vi "UpdateCfgIni.vi"(8 "error in":errorcluster, 10 "contentArray":string[](array[string]), 11 "iniCfgRefnumIn":refnum<file>) -> (0 "error out":errorcluster, 3 "iniCfgRefnumOut":refnum<file>)   [LabVIEW 2010]
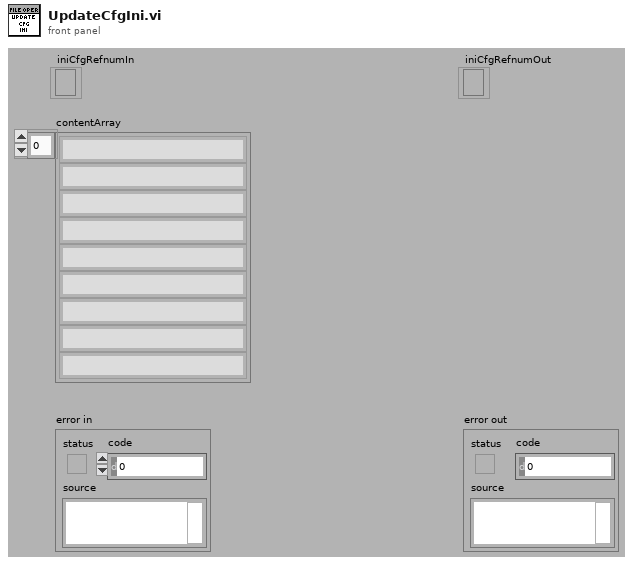
[diagram p1: front panel]
types:
  T1 = enum16{"open", "replace", "create", "open or create", "replace or create", "replace or create with confirmation"}
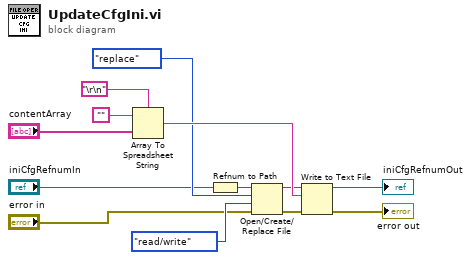
[diagram p0: block diagram]
diagram:
  n1 = Array To Spreadsheet String(delimiter (Tab)="\r\n", array="contentArray", 3:"") -> (spreadsheet string=w10:string)
  n2 = Refnum to Path(1:"iniCfgRefnumIn") -> (0:w6:path)
  n3 = Open/Create/Replace File(file path (use dialog)=w6, error in="error in", operation (0:open)=T1."replace", access (0:read/write)=enum16{"read/write", "read-only", "write-only"}."read/write") -> (refnum out=w9:refnum<file>, error out=w11:errorcluster)  [unwired: 2 in, 1 out]
  n4 = Write to Text File(file (use dialog)=w9, text=w10, error in=w11) -> (refnum out=→"iniCfgRefnumOut":refnum<file>, error out=→"error out":errorcluster)  [unwired: 1 in, 1 out]
